vi "reg-io-conf.vi"(9 "menu (List Configs)":T6=enum."IO List Configs", 10 "Key":string, 11 "IO Node in":T1={"ADDR"=203, "Label"="CLMX_Tdry", "Type"=enum."AI", "Mode"=enum."RIO", "Value"="-128.47", "Tags"="", "calibration"=[{"X"=1600.0, "Y"=1.0}, {"X"=1800.0, "Y"=22.0}]} {"calibration"."Y" format="%#.3f"; "calibration"."X" format="%#.3f"; "ADDR" format="%04d"}) -> (1 "Key Not Found?":bool, 2 "List Nodes":T1[](array[typedef]) {"calibration"."Y" format="%#.3f"; "calibration"."X" format="%#.3f"; "ADDR" format="%04d"}, 3 "IO Node out":T1={"ADDR"=203, "Label"="CLMX_Tdry", "Type"=enum."AI", "Mode"=enum."RIO", "Value"="-128.47", "Tags"="", "calibration"=[{"X"=1600.0, "Y"=1.0}, {"X"=1800.0, "Y"=22.0}]} {"calibration"."Y" format="%#.3f"; "calibration"."X" format="%#.3f"; "ADDR" format="%04d"})   [LabVIEW 2024]
doc: "This VI demonstrates basic use of the map data type. Maps are used to create a collection of keys and associate each unique key with a value. The user selects the two data types used for the keys and for the values.\n\nThis example uses maps to count the occurrences of each word within a block of text."
uses:
  controls/IONode.ctl
  controls/type.address.ctl
  controls/enum.io.type.ctl
  controls/enum.io.mode.ctl
  controls/typeXyPoint.ctl
  controls/enumVarCtrlIO.ctl
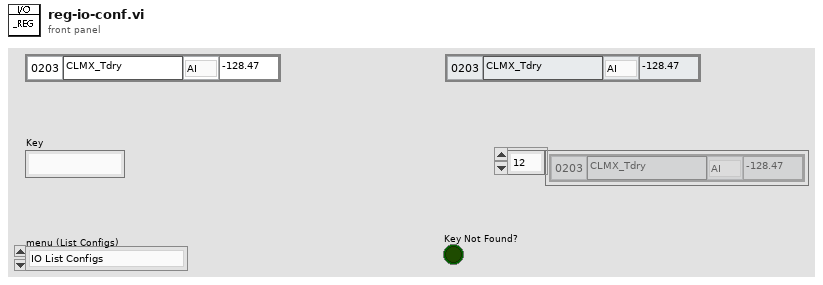
[diagram p1: front panel]
types:
  T1 = typedef "IONode.ctl" = cluster{"ADDR":T2, "Label":string, "Type":T3, "Mode":T4, "Value":string, "Tags":string, "calibration":T5[]}
  T2 = typedef "type.address.ctl" = u16
  T3 = typedef "enum.io.type.ctl" = enum16{"Type", "DI", "DO", "AI", "AO", "VL", "BUF"}
  T4 = typedef "enum.io.mode.ctl" = enum16{"Mode", "RIO", "SIM"}
  T5 = typedef "typeXyPoint.ctl" = cluster{"X":dbl, "Y":dbl}
  T6 = typedef "enumVarCtrlIO.ctl" = enum16{"IO Get By Key", "IO List Configs", "IO Add By Key", "IO Modify Value By Key", "IO Modify Calib By Key", "IO Modify ADDR By Key", "IO Modify Mode By Key", "IO Modify Type By Key", "IO Modify Name By Key", "IO Remove By Key", "IO Remove All"}
  T7 = enum32{"Modify Entry only if found", "Add or Modify Entry", "Delete Entry"}
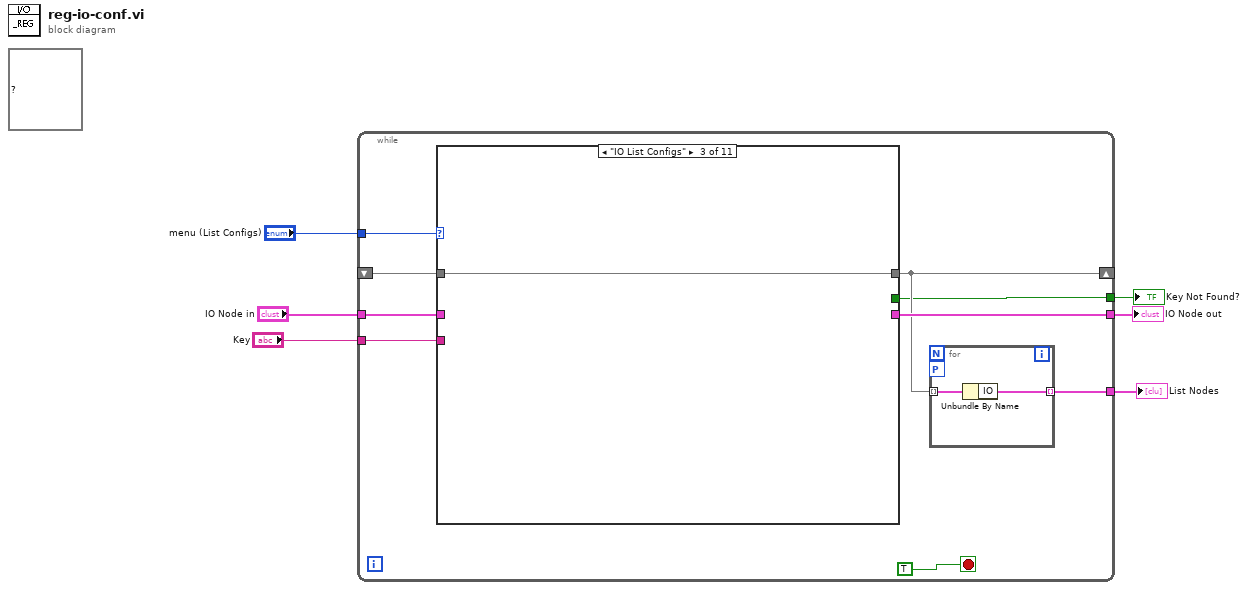
[diagram p0: block diagram]
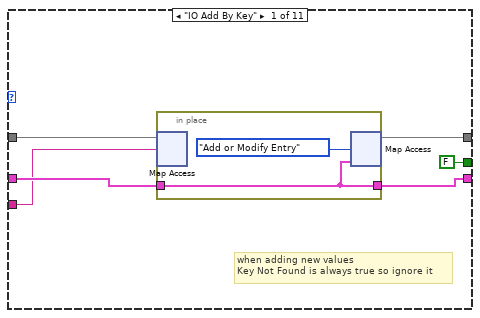
[diagram p2: hidden frame]
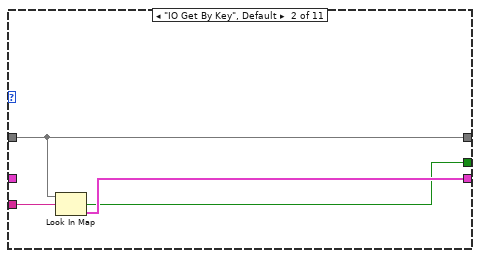
[diagram p3: hidden frame]
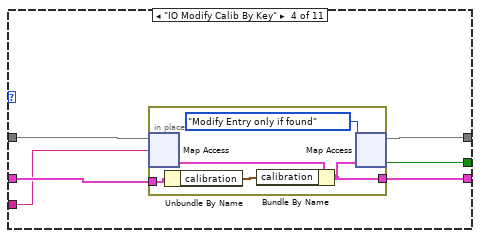
[diagram p4: hidden frame]
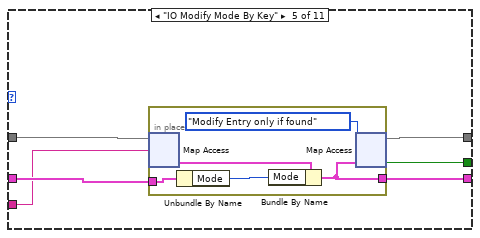
[diagram p5: hidden frame]
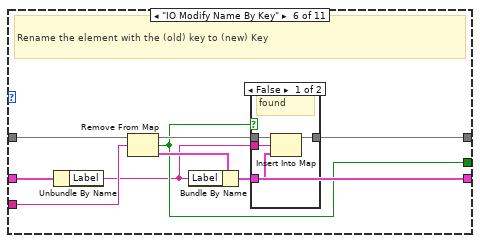
[diagram p6: hidden frame]
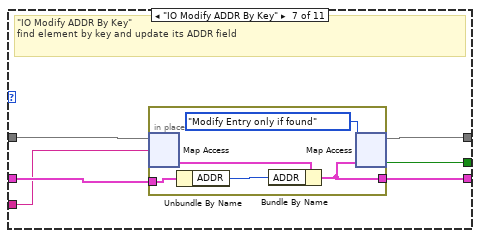
[diagram p8: hidden frame]
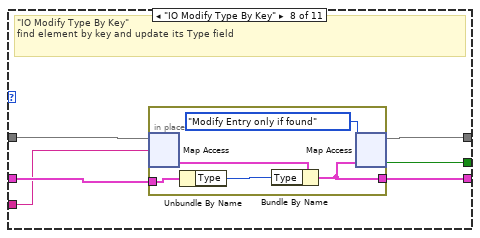
[diagram p9: hidden frame]
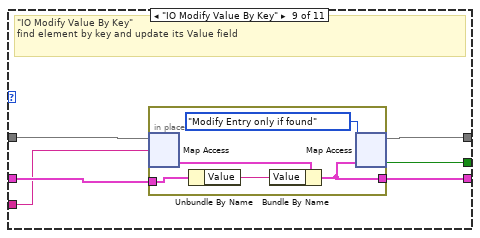
[diagram p10: hidden frame]
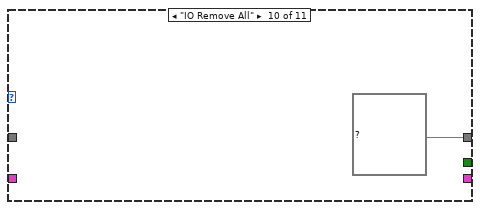
[diagram p11: hidden frame]
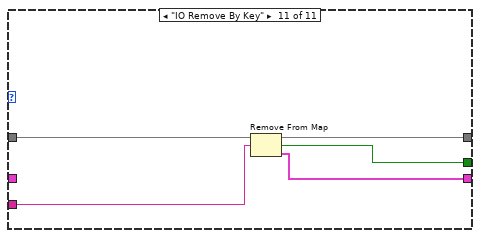
[diagram p12: hidden frame]
diagram:
  (unwired) map{string, T1} {} ("map constant")
  n1 = while {
    tunnel: "menu (List Configs)" -> [w15]
    shift-right: [w8] -> _
    shift-left: _ -> [w14]
    tunnel: "IO Node in" -> [w12]
    tunnel: [w7] -> w4
    tunnel: [w11] -> w3
    tunnel: [w9] -> w2
    tunnel: "Key" -> [w10]
    stop <- TRUE ("stop") stop-if-true
    n2 = case shown="\"IO List Configs\"" w15 {
      tunnel: [w23 w29 w30 w36 w47 w59 w72 w83 w94 map{string, T1} {} ("map constant") w104] -> w8
      tunnel: w14 -> [w22 w29 w30 w35 w46 w61 w71 w82 w93 _ w105]
      tunnel: w12 -> [w21 _ _ w34 w45 w56 w70 w81 w92 _ _]
      tunnel: [w20 w28 _ w33 w44 w57 w69 w80 w91 _ w103] -> w11
      tunnel: w10 -> [w19 w27 _ w32 w43 w54 w68 w79 w90 _ w102]
      tunnel: [FALSE ("key not found?") w26 _ w31 w42 w55 w67 w78 w89 _ w101] -> w7
      frame "IO Add By Key" {
        (unwired) FALSE ("key not found?")
        (unwired) FALSE ("key not found?")
        # "when adding new values \nKey Not Found is always true so ignore it"
        n3 = in-place {
          in-place-border: w21 -> [w24]
          in-place-border: [w24] -> w20
          n4 = in-place-map #1(w22, w19) -> ()  [unwired: 1 in, 2 out]
          n5 = in-place-map #1(w24, T7."Add or Modify Entry" ("action")) -> (w23:map{string, T1})  [unwired: 2 out]
        }
      }
      frame "IO Get By Key", Default {
        n6 = Look In Map(map=w29, key=w27) -> (key not found?=w26:bool, value=w28:T1)  [unwired: 1 in]
      }
      frame "IO List Configs" {
      }
      frame "IO Modify Calib By Key" {
        n7 = in-place {
          in-place-border: w34 -> [w38]
          in-place-border: [w39] -> w33
          n8 = in-place-map #2(w35, w32) -> (w40:T1)  [unwired: 1 in, 1 out]
          n9 = Unbundle By Name(w38) -> ("calibration"=w37:T5[])
          n10 = Bundle By Name(cluster=w40, "calibration"=w37) -> (w39:T1)
          n11 = in-place-map #2(w39, T7."Modify Entry only if found" ("action")) -> (w36:map{string, T1}, w31:bool)  [unwired: 1 out]
        }
      }
      frame "IO Modify Mode By Key" {
        n12 = in-place {
          in-place-border: w45 -> [w49]
          in-place-border: [w50] -> w44
          n13 = in-place-map #3(w46, w43) -> (w51:T1)  [unwired: 1 in, 1 out]
          n14 = Unbundle By Name(w49) -> ("Mode"=w48:T4)
          n15 = Bundle By Name(cluster=w51, "Mode"=w48) -> (w50:T1)
          n16 = in-place-map #3(w50, T7."Modify Entry only if found" ("action")) -> (w47:map{string, T1}, w42:bool)  [unwired: 1 out]
        }
      }
      frame "IO Modify Name By Key" {
        # "Rename the element with the (old) key to (new) Key"
        n17 = Unbundle By Name(w56) -> ("Label"=w53:string)
        n18 = Remove From Map(10:w54, 11:w61) -> (1:w58:T1, 2:w55:bool, 3:w60:map{string, T1})
        n19 = Bundle By Name(cluster=w58, "Label"=w53) -> (w57:T1)
        n20 = case shown="False" w55 {
          tunnel: w60 -> [w65 w66]
          tunnel: [w64 w66] -> w59
          tunnel: w57 -> [w63 _]
          tunnel: w53 -> [w62 _]
          frame False {
            # "found"
            n21 = Insert Into Map(map in=w65, key=w62, value=w63) -> (map out=w64:map{string, T1})  [unwired: 2 out]
          }
          frame True {
            # "not found"
          }
        }
      }
      frame "IO Modify ADDR By Key" {
        # "\"IO Modify ADDR By Key\"  \nfind element by key and update its ADDR field"
        n22 = in-place {
          in-place-border: w70 -> [w74]
          in-place-border: [w75] -> w69
          n23 = in-place-map #4(w71, w68) -> (w76:T1)  [unwired: 1 in, 1 out]
          n24 = Unbundle By Name(w74) -> ("ADDR"=w73:T2)
          n25 = Bundle By Name(cluster=w76, "ADDR"=w73) -> (w75:T1)
          n26 = in-place-map #4(w75, T7."Modify Entry only if found" ("action")) -> (w72:map{string, T1}, w67:bool)  [unwired: 1 out]
        }
      }
      frame "IO Modify Type By Key" {
        # "\"IO Modify Type By Key\"\nfind element by key and update its Type field"
        n27 = in-place {
          in-place-border: w81 -> [w85]
          in-place-border: [w86] -> w80
          n28 = in-place-map #5(w82, w79) -> (w87:T1)  [unwired: 1 in, 1 out]
          n29 = Unbundle By Name(w85) -> ("Type"=w84:T3)
          n30 = Bundle By Name(cluster=w87, "Type"=w84) -> (w86:T1)
          n31 = in-place-map #5(w86, T7."Modify Entry only if found" ("action")) -> (w83:map{string, T1}, w78:bool)  [unwired: 1 out]
        }
      }
      frame "IO Modify Value By Key" {
        # "\"IO Modify Value By Key\" \nfind element by key and update its Value field"
        n32 = in-place {
          in-place-border: w92 -> [w96]
          in-place-border: [w97] -> w91
          n33 = in-place-map #6(w93, w90) -> (w98:T1)  [unwired: 1 in, 1 out]
          n34 = Unbundle By Name(w96) -> ("Value"=w95:string)
          n35 = Bundle By Name(cluster=w98, "Value"=w95) -> (w97:T1)
          n36 = in-place-map #6(w97, T7."Modify Entry only if found" ("action")) -> (w94:map{string, T1}, w89:bool)  [unwired: 1 out]
        }
      }
      frame "IO Remove All" {
      }
      frame "IO Remove By Key" {
        n37 = Remove From Map(10:w102, 11:w105) -> (1:w103:T1, 2:w101:bool, 3:w104:map{string, T1})
      }
    }
    n38 = for {
      tunnel: w8 -> [w17] mode=indexing
      tunnel: [w16] -> w9 mode=indexing
      workers-P: _ -> [_]
      n39 = Unbundle By Name(w17) -> ("IO"=w16:T1)
    }
  }
  "Key Not Found?" <- w4
  "IO Node out" <- w3
  "List Nodes" <- w2
